vi "ValvulaUnitáriaV18.vi"() -> ()   [LabVIEW 2019]
uses:
  <vilib>/DAQmx/read.llb/DAQmx Read (Analog 1D DBL NChan 1Samp).vi
  <vilib>/DAQmx/read.llb/DAQmx Read (Analog 2D DBL NChan NSamp).vi
  <vilib>/DAQmx/create/channels.llb/DAQmx Create Channel (CO-Pulse Generation-Frequency).vi
  <vilib>/DAQmx/configure/timing.llb/DAQmx Timing (Implicit).vi
  <vilib>/DAQmx/configure/timing.llb/DAQmx Timing (Sample Clock).vi
  <vilib>/DAQmx/miscellaneous.llb/DAQmx Fill In Error Info.vi
  <vilib>/Analysis/NI_AALBase.lvlib
  <vilib>/Analysis/baseanly.llb/Mean (DBL).vi
  <resource>/objmgr/daqmx.rc
panel:
  out "Return from 0":bool
  out "Permanent regime":bool
  out "Samples saved":i32
  in  "Automático":bool
  in  "Duty Cycle %":dbl=50.0 min=5.0 max=50.0 step=1.0
  in  "Valvula 2":bool=TRUE
  in  "resetDaq":bool
  out "DAQ Rate":i32=100 min=1 max=10000 step=1
  in  "Samples per Cycle":i32=200 min=1 max=100000 step=1
  out "Motor stopping":bool
  out "Motor working":bool
  in  "Frequency":dbl=1.0 min=0.8 max=8.0 step=0.1
  out "CAME Frequency":dbl
  in  "Start Motor":bool
  out "StepMotorValueChanged":bool
  out "Cycles":i32
  in  "File Name":string="test"
  in  "?":enum32{"Page 1", "Page 2"}(tab)
  out "Torque":dbl(graph)
  out "Valve state signal":dbl[][](graph)
  out "Flowrate":dbl(graph)
  out "Pressures":dbl[][](graph)
  out "Displacements":dbl[][](graph)
  out "Indutive Sensor":dbl(graph)
  in  "Save aquisition":bool
  in  "File Path":path=path "G:/My Drive/MagChill/Sistema Hidráulico/6.Dados_Testes/2.Etapa_ii"
  in  "Stop":bool
  out "Stop operations":bool
  # "File Path"
  # "File name:"
  # "Eletrovalve/CAME\n       Frequency"
  # "Samples per Cycles"
  # "DAQ Rate"
  # "Cycles"
  # "Samples Saved"
  # "Write to File"
  # "Stop Program"
  # "CAME Operation"
  # "Start/Stop Motor\n(operation cycle)"
  # "CAME Frequency"
  # "Eletrovalve Operation"
  # "Start/Stop Eletrovalve\n     (operation cycle)"
  # "% Duty Cycle"
  # "On/Off Manual"
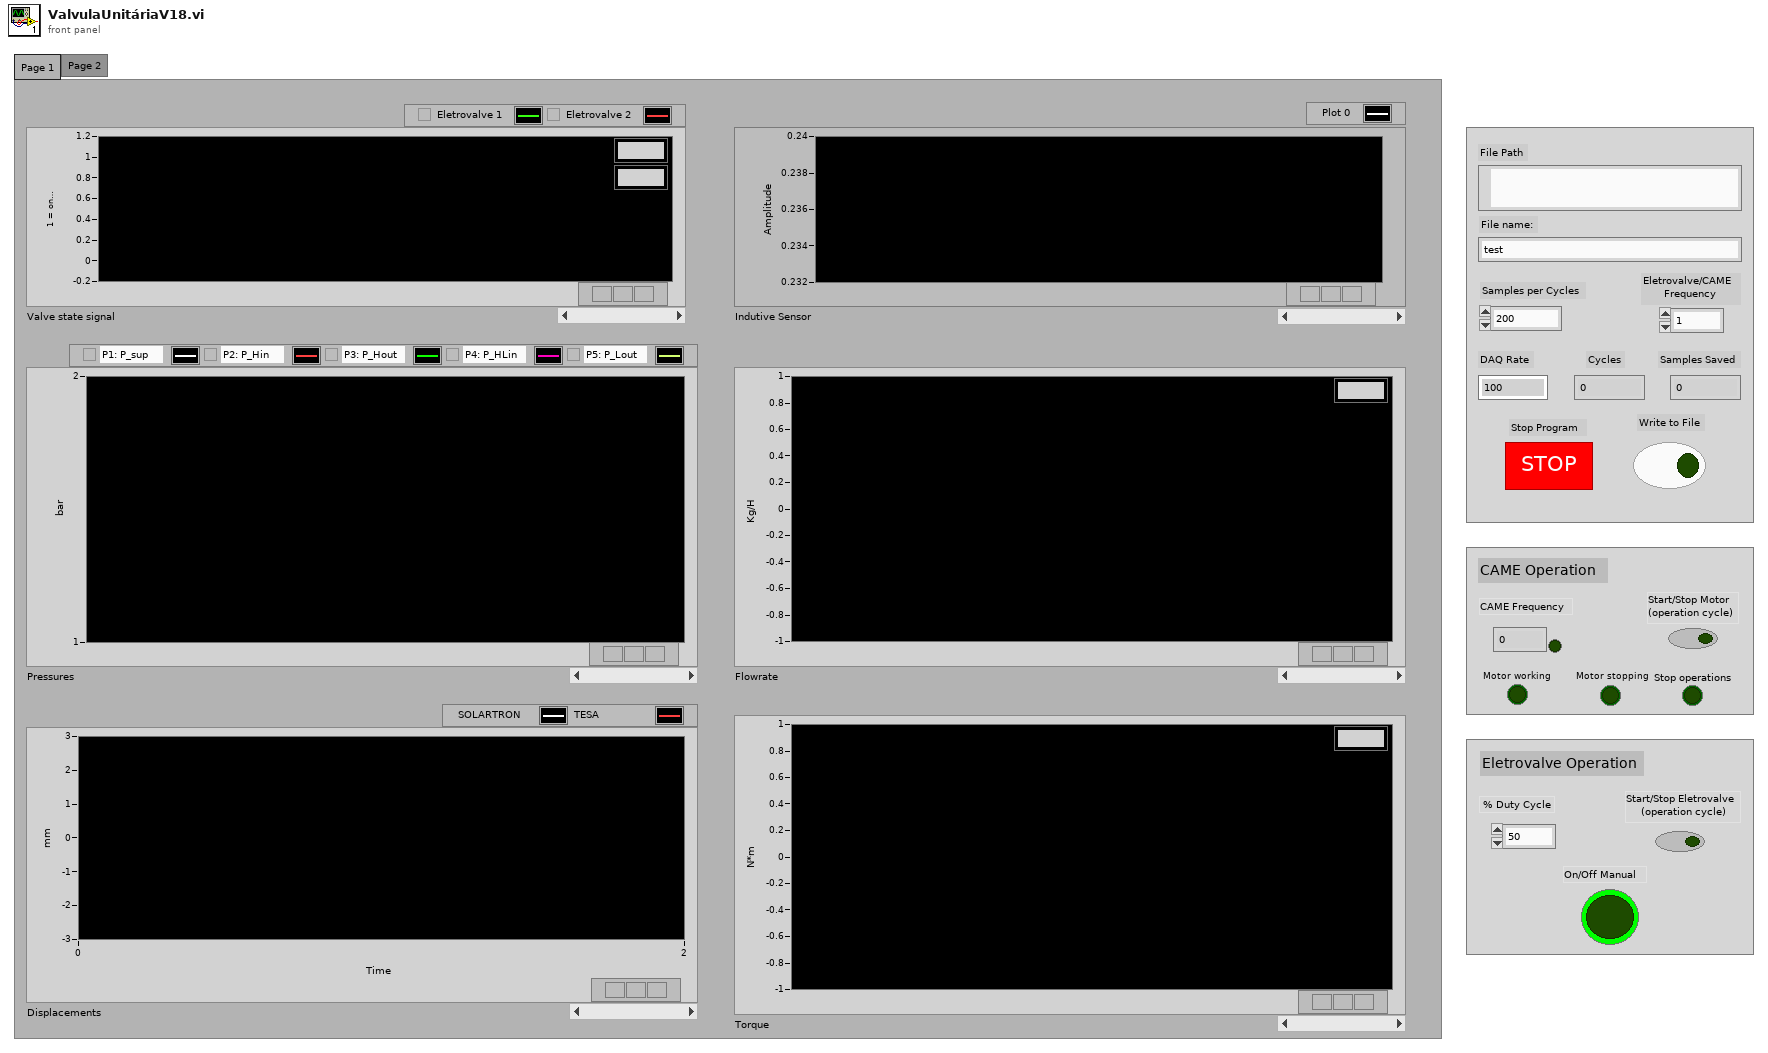
[diagram p1: front panel]
types:
  T1 = enum8{"Enabled", "Disabled", "Disabled and Grayed Out"}
  T2 = enum16{"open", "open or create", "create or replace", "create", "open (read only)"}
  T3 = cluster{"Automatico":bool, "Valvula":bool, "Duty cycle":dbl, "Stop":bool, "Frequencia":dbl}
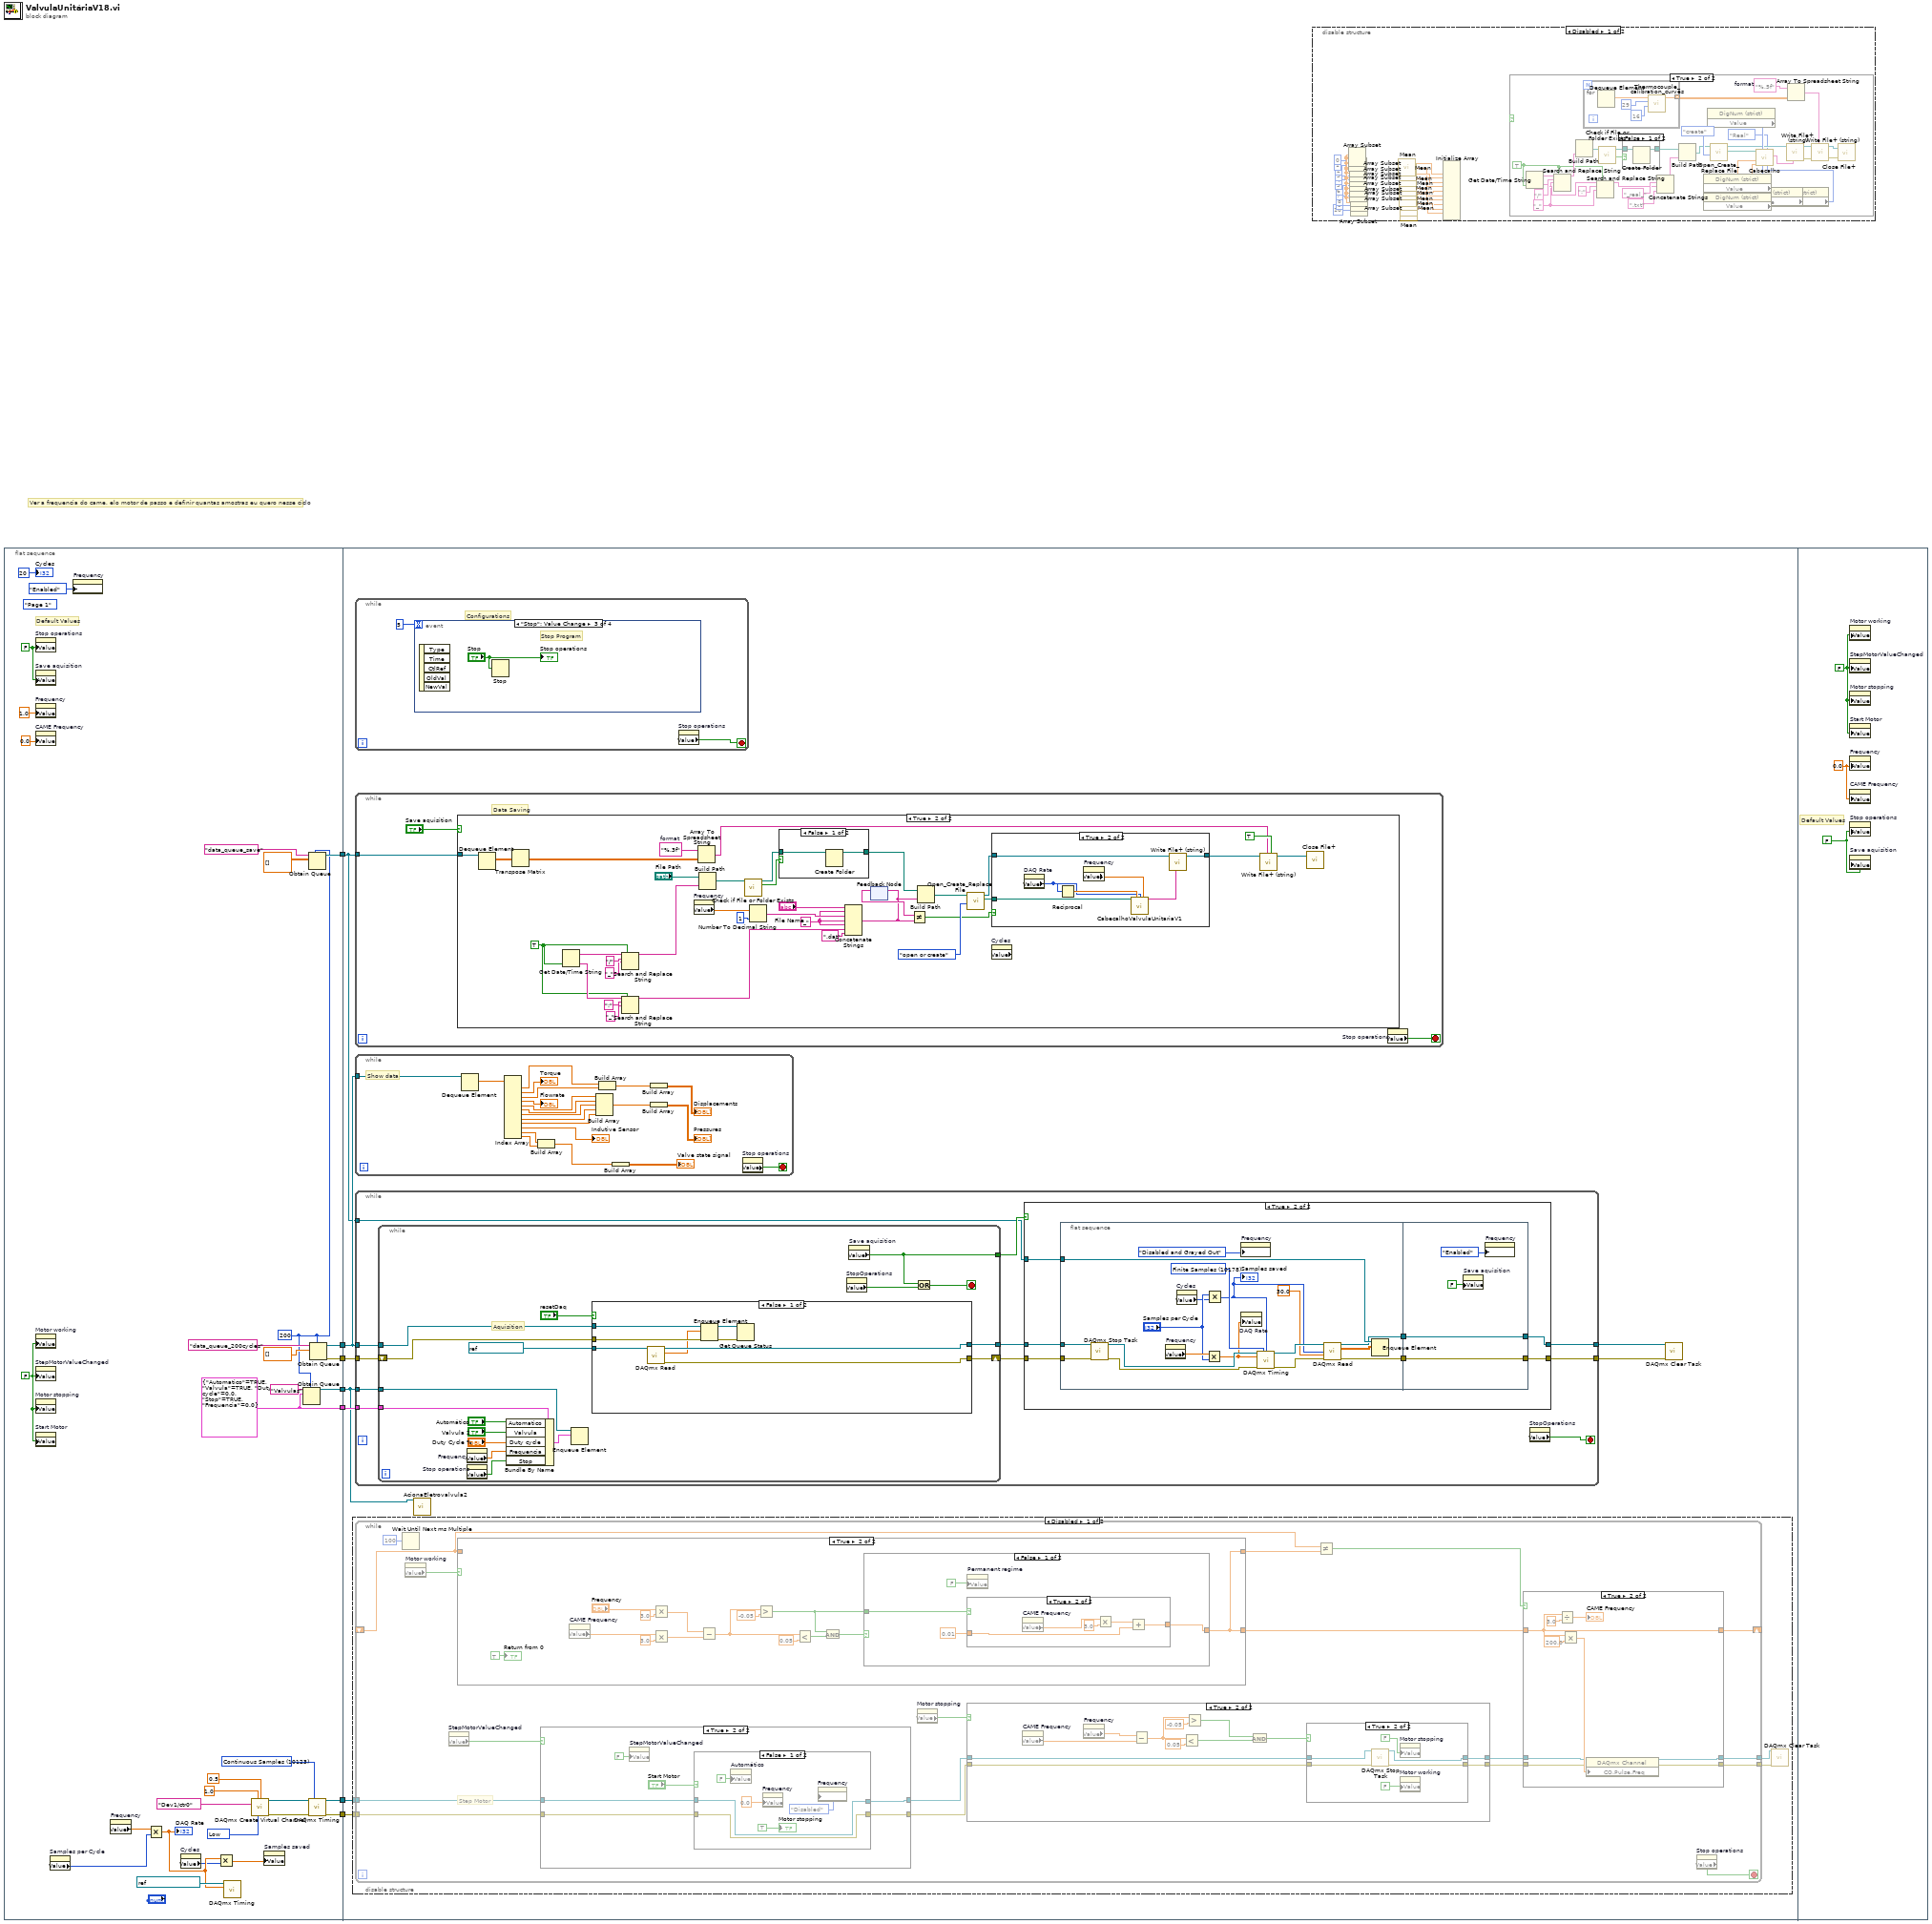
[diagram p0: block diagram]
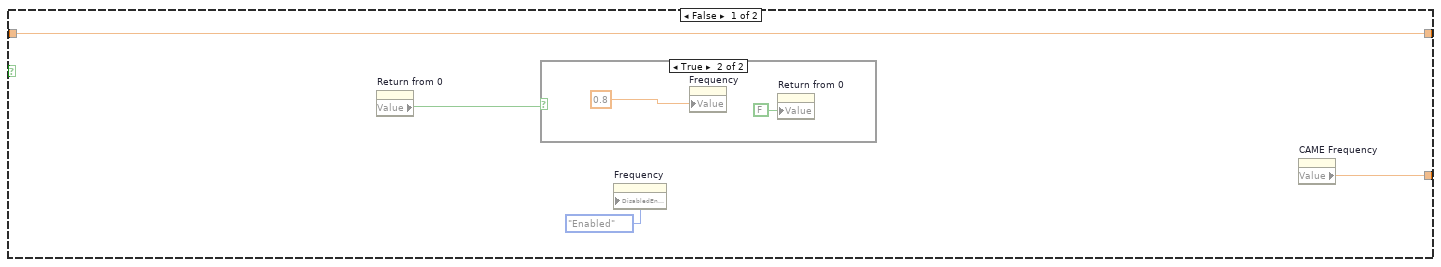
[diagram p4: hidden frame]
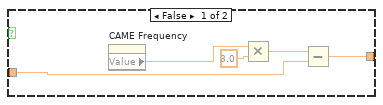
[diagram p6: hidden frame]
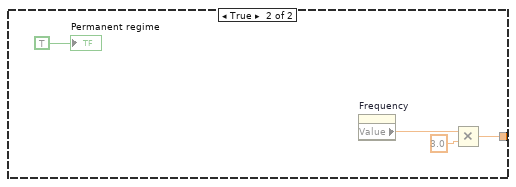
[diagram p7: hidden frame]
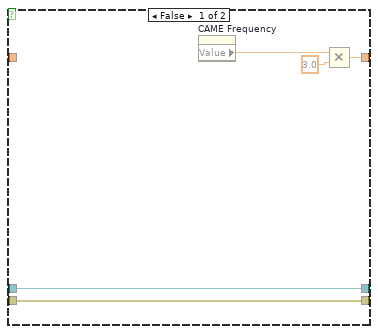
[diagram p8: hidden frame]
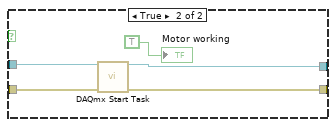
[diagram p10: hidden frame]
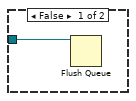
[diagram p12: hidden frame]
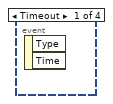
[diagram p15: hidden frame]
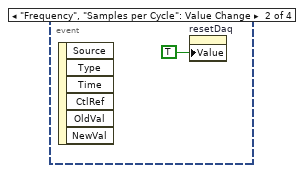
[diagram p16: hidden frame]
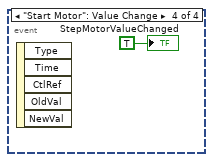
[diagram p17: hidden frame]
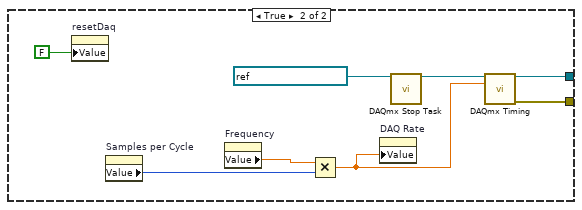
[diagram p19: hidden frame]
diagram:
  # "Ver a frequencia do came, elo motor de passo e definir quantas amostras eu quero nesse ciclo"
  n1 = flat-sequence {
    tunnel: [w39] -> w7
    tunnel: [w37] -> w6
    tunnel: [w28] -> w5
    tunnel: [w29] -> w4
    tunnel: [w24] -> w3
    tunnel: [w11] -> w2
    tunnel: [w10] -> w1
    tunnel: w7 -> [w43]
    tunnel: w6 -> [w48]
    tunnel: w5 -> [w46]
    tunnel: w4 -> [w47]
    tunnel: w3 -> [w42]
    tunnel: w2 -> [w40]
    tunnel: w1 -> [w41]
    frame #0 {
      w10 = T3 {"Automatico"=TRUE, "Valvula"=TRUE, "Duty cycle"=0.0, "Stop"=TRUE, "Frequencia"=0.0}
      w9 = 200 ("max queue size (-1, unlimited)")
      w26 = FALSE ("RestartOperations")
      w27 = FALSE
      w34 = 10123 items=["Finite Samples"=10178, "Continuous Samples"=10123, "Hardware Timed Single Point"=12522] ("sample mode")
      w30 = 10214 items=["High"=10192, "Low"=10214] ("idle state")
      (unwired) enum32{"Page 1", "Page 2"}."Page 1" ("Tab Control")
      # "Default Values"
      n2 = property on="Stop operations" class="Bool (strict)"("Value"=w26) -> ()  [unwired: 2 in, 2 out]
      n3 = property on="Save aquisition" class="Bool (strict)"("Value"=w26) -> ()  [unwired: 2 in, 2 out]
      n4 = property on="Frequency" class="DigNum (strict)"("Value"=1.0 ("SP CAME Frequency")) -> ()  [unwired: 2 in, 2 out]
      n5 = property on="CAME Frequency" class="DigNum (strict)"("Value"=0.0 ("CAME Frequency")) -> ()  [unwired: 2 in, 2 out]
      n6 = property on="Motor working" class="Bool (strict)"("Value"=w27) -> ()  [unwired: 2 in, 2 out]
      n7 = property on="StepMotorValueChanged" class="Bool (strict)"("Value"=w27) -> ()  [unwired: 2 in, 2 out]
      n8 = property on="Motor stopping" class="Bool (strict)"("Value"=w27) -> ()  [unwired: 2 in, 2 out]
      n9 = property on="Start Motor" class="Bool (strict)"("Value"=w27) -> ()  [unwired: 2 in, 2 out]
      n10 = property on="Samples per Cycle" class="DigNum (strict)"() -> ("Value"=w17:i32)  [unwired: 2 in, 2 out]
      n11 = property on="Frequency" class="DigNum (strict)"("DisabledEnum"=T1."Enabled" ("Disabled")) -> ()  [unwired: 2 in, 2 out]
      n12 = property on="Frequency" class="DigNum (strict)"() -> ("Value"=w21:dbl)  [unwired: 2 in, 2 out]
      n13 = Multiply(x=w21, y=w17) -> (x*y=w15:dbl)
      "DAQ Rate" <- w15
      n14 = property on="Cycles" class="DigNum (strict)"() -> ("Value"=w14:i32)  [unwired: 2 in, 2 out]
      n15 = Multiply(x=w15, y=w14) -> (x*y=w13:dbl)
      n16 = call-poly <vilib>:"DAQmx Timing.vi"("task/channels in"=refnum<k21> "AnalogInputs", "rate"=w15) -> ()  [unwired: 12 in, 2 out]
      n17 = call-poly <vilib>:"DAQmx Create Virtual Channel.vi"("frequency"=1.0, "duty cycle"=0.5, "counter"=tag "Dev1/ctr0", "idle state"=w30) -> ("task out"=w36:refnum<k21>, "error out"=w35:errorcluster)  [unwired: 10 in]
      n18 = property on="Samples saved" class="DigNum (strict)"("Value"=w13) -> ()  [unwired: 2 in, 2 out]
      n19 = Obtain Queue(max queue size (-1, unlimited)=w9, name (unnamed)="Valvulas", element data type=w10) -> (queue out=w11:refnum<queue>)  [unwired: 2 in, 2 out]
      n20 = Obtain Queue(max queue size (-1, unlimited)=w9, name (unnamed)="data_queue_save", element data type=dbl[][] [] ("data")) -> (queue out=w24:refnum<queue>)  [unwired: 2 in, 2 out]
      n21 = call-poly <vilib>:"DAQmx Timing.vi"("task/channels in"=w36, "sample mode"=w34, "error in"=w35) -> ("task out"=w29:refnum<k21>, "error out"=w28:errorcluster)  [unwired: 11 in]
      n22 = Obtain Queue(max queue size (-1, unlimited)=w9, name (unnamed)="data_queue_200cycles", element data type=dbl[] [] ("data")) -> (queue out=w39:refnum<queue>, error out=w37:errorcluster)  [unwired: 2 in, 1 out]
      "Cycles" <- 20 ("Cycles")
    }
    frame #1 {
      n23 = disable-structure shown="Disabled" {
        disable-tunnel: w47 -> [w52 _]
        disable-tunnel: w46 -> [w51 _]
        frame Disabled {
          n24 = while {
            tunnel: w52 -> [w70]
            tunnel: w51 -> [w69]
            shift-right: [w67] -> _
            shift-left: _ -> [w63]
            tunnel: [w55] -> w50
            tunnel: [w54] -> w49
            stop <- w53 stop-if-true
            # "Step Motor"
            n25 = Wait Until Next ms Multiple(millisecond multiple=u32 100) -> ()  [unwired: 1 out]
            n26 = property on="Motor working" class="Bool (strict)"() -> ("Value"=w66:bool)  [unwired: 2 in, 2 out]
            n27 = property on="StepMotorValueChanged" class="Bool (strict)"() -> ("Value"=w68:bool)  [unwired: 2 in, 2 out]
            n28 = case shown="True" w66 {
              tunnel: w63 -> [w96 _]
              tunnel: [w95 w108] -> w57
              tunnel: [w96 w108] -> w65
              frame False {
                n29 = property on="Return from 0" class="Bool (strict)"() -> ("Value"=w93:bool)  [unwired: 2 in, 2 out]
                n30 = case shown="True" w93 {
                  frame False {
                  }
                  frame True {
                    n31 = property on="Frequency" class="DigNum (strict)"("Value"=0.8 ("SP Frequency")) -> ()  [unwired: 2 in, 2 out]
                    n32 = property on="Return from 0" class="Bool (strict)"("Value"=FALSE ("Return from 0")) -> ()  [unwired: 2 in, 2 out]
                  }
                }
                n33 = property on="Frequency" class="DigNum (strict)"("DisabledEnum"=T1."Enabled" ("Disabled")) -> ()  [unwired: 2 in, 2 out]
                n34 = property on="CAME Frequency" class="DigNum (strict)"() -> ("Value"=w95:dbl)  [unwired: 2 in, 2 out]
              }
              frame True {
                n35 = property on="CAME Frequency" class="DigNum (strict)"() -> ("Value"=w103:dbl)  [unwired: 2 in, 2 out]
                n36 = Multiply(x="Frequency", y=3.0) -> (x*y=w104:dbl)
                n37 = Multiply(x=w103, y=3.0) -> (x*y=w101:dbl)
                n38 = Subtract(x=w104, y=w101) -> (x-y=w106:dbl)
                n39 = Greater?(x=w106, y=-0.05) -> (0:w107:bool)
                n40 = Less?(x=w106, y=0.05) -> (x < y?=w110:bool)
                n41 = And(x=w107, y=w110) -> (x .and. y?=w109:bool)
                n42 = case shown="False" w109 {
                  tunnel: [w115 w130] -> w108
                  tunnel: w107 -> [w116 _]
                  frame False {
                    n43 = property on="Permanent regime" class="Bool (strict)"("Value"=FALSE ("Permanent regime")) -> ()  [unwired: 2 in, 2 out]
                    n44 = case shown="True" w116 {
                      tunnel: [w121 w126] -> w115
                      tunnel: 0.01 ("y") -> [w120 w125]
                      frame False {
                        n45 = property on="CAME Frequency" class="DigNum (strict)"() -> ("Value"=w119:dbl)  [unwired: 2 in, 2 out]
                        n46 = Multiply(x=w119, y=3.0) -> (x*y=w117:dbl)
                        n47 = Subtract(x=w117, y=w120) -> (x-y=w121:dbl)
                      }
                      frame True {
                        n48 = property on="CAME Frequency" class="DigNum (strict)"() -> ("Value"=w124:dbl)  [unwired: 2 in, 2 out]
                        n49 = Multiply(x=w124, y=3.0) -> (x*y=w122:dbl)
                        n50 = Add(x=w122, y=w125) -> (x+y=w126:dbl)
                      }
                    }
                  }
                  frame True {
                    n51 = property on="Frequency" class="DigNum (strict)"() -> ("Value"=w129:dbl)  [unwired: 2 in, 2 out]
                    n52 = Multiply(x=w129, y=3.0) -> (x*y=w130:dbl)
                    "Permanent regime" <- TRUE ("Permanent regime")
                  }
                }
                "Return from 0" <- TRUE ("Return from 0")
              }
            }
            n53 = case shown="True" w68 {
              tunnel: w70 -> [w146 w151]
              tunnel: w69 -> [w145 w150]
              tunnel: [w146 w147] -> w61
              tunnel: [w145 w152] -> w60
              frame False {
              }
              frame True {
                n54 = property on="StepMotorValueChanged" class="Bool (strict)"("Value"=FALSE) -> ()  [unwired: 2 in, 2 out]
                n55 = case shown="False" "Start Motor" {
                  tunnel: [w157 w163] -> w147
                  tunnel: [w156 w162] -> w152
                  tunnel: w151 -> [w157 w161]
                  tunnel: w150 -> [w156 w160]
                  frame False {
                    n56 = property on="Automático" class="Bool (strict)"("Value"=FALSE ("Automático")) -> ()  [unwired: 2 in, 2 out]
                    n57 = property on="Frequency" class="DigNum (strict)"("Value"=0.0 ("SP Frequency")) -> ()  [unwired: 2 in, 2 out]
                    n58 = property on="Frequency" class="DigNum (strict)"("DisabledEnum"=T1."Disabled" ("Disabled")) -> ()  [unwired: 2 in, 2 out]
                    "Motor stopping" <- TRUE ("Motor stopping")
                  }
                  frame True {
                    n59 = call <vilib>:"DAQmx Start Task.vi"("task/channels in"=w161, "error in"=w160) -> ("task out"=w163:refnum<k21>, "error out"=w162:errorcluster)  [unwired: 12 in]
                    "Motor working" <- TRUE ("Motor working")
                  }
                }
              }
            }
            n60 = property on="Motor stopping" class="Bool (strict)"() -> ("Value"=w62:bool)  [unwired: 2 in, 2 out]
            n61 = case shown="True" w62 {
              tunnel: w61 -> [w72 w78]
              tunnel: w60 -> [w71 w77]
              tunnel: [w72 w76] -> w59
              tunnel: [w71 w75] -> w58
              frame False {
              }
              frame True {
                n62 = property on="CAME Frequency" class="DigNum (strict)"() -> ("Value"=w73:dbl)  [unwired: 2 in, 2 out]
                n63 = property on="Frequency" class="DigNum (strict)"() -> ("Value"=w80:dbl)  [unwired: 2 in, 2 out]
                n64 = Subtract(x=w80, y=w73) -> (x-y=w83:dbl)
                n65 = Less?(x=w83, y=0.05) -> (x < y?=w82:bool)
                n66 = Greater?(x=w83, y=-0.05) -> (0:w81:bool)
                n67 = And(x=w81, y=w82) -> (x .and. y?=w79:bool)
                n68 = case shown="True" w79 {
                  tunnel: w78 -> [w86 w92]
                  tunnel: w77 -> [w85 w91]
                  tunnel: [w86 w90] -> w76
                  tunnel: [w85 w89] -> w75
                  frame False {
                  }
                  frame True {
                    n69 = call <vilib>:"DAQmx Stop Task.vi"("task/channels in"=w92, "error in"=w91) -> ("task out"=w90:refnum<k21>, "error out"=w89:errorcluster)  [unwired: 12 in]
                    n70 = property on="Motor stopping" class="Bool (strict)"("Value"=FALSE ("Motor stopping")) -> ()  [unwired: 2 in, 2 out]
                    n71 = property on="Motor working" class="Bool (strict)"("Value"=FALSE ("Motor working")) -> ()  [unwired: 2 in, 2 out]
                  }
                }
              }
            }
            n72 = Not Equal?(x=w63, y=w65) -> (x != y?=w64:bool)
            n73 = case shown="True" w64 {
              tunnel: [w135 w144] -> w55
              tunnel: [w134 w143] -> w54
              tunnel: w57 -> [_ w137]
              tunnel: [w131 w137] -> w67
              tunnel: w59 -> [w135 w140]
              tunnel: w58 -> [w134 w139]
              frame False {
                n74 = property on="CAME Frequency" class="DigNum (strict)"() -> ("Value"=w133:dbl)  [unwired: 2 in, 2 out]
                n75 = Multiply(x=w133, y=3.0) -> (x*y=w131:dbl)
              }
              frame True {
                n76 = Divide(x=w137, y=3.0) -> (x/y=→"CAME Frequency":dbl)
                n77 = Multiply(x=w137, y=200.0) -> (x*y=w141:dbl)
                n78 = property class="DAQmx Channel"(reference=w140, error in=w139, "CO.Pulse.Freq"=w141) -> (reference out=w144:refnum<k21>, error out=w143:errorcluster)
              }
            }
            n79 = property on="Stop operations" class="Bool (strict)"() -> ("Value"=w53:bool)  [unwired: 2 in, 2 out]
          }
          n80 = call <vilib>:"DAQmx Clear Task.vi"("task in"=w50, "error in"=w49) -> ()  [unwired: 13 in, 1 out]
        }
        frame Enabled {
        }
      }
      n81 = while {
        stop <- w235 stop-if-true
        # "Configurations"
        n82 = event shown="[2] \"Stop\": Value Change" {
          selector: _ -> [_ _ _ _]
          dyn-events: _ -> [_ _ _ _]
          timeout: 5 -> [_ _ _ _]
          event Timeout {
            n83 = event-data() -> ()  [unwired: 1 in, 2 out]
          }
          event "Frequency", "Samples per Cycle": Value Change {
            n84 = event-data() -> ()  [unwired: 1 in, 6 out]
            n85 = property on="resetDaq" class="Bool (strict)"("Value"=TRUE ("resetDaq")) -> ()  [unwired: 2 in, 2 out]
          }
          event "Stop": Value Change {
            # "Stop Program"
            n86 = event-data() -> ()  [unwired: 1 in, 5 out]
            n87 = Stop(stop? (T)="Stop") -> ()
            "Stop operations" <- "Stop"
          }
          event "Start Motor": Value Change {
            n88 = event-data() -> ()  [unwired: 1 in, 5 out]
            "StepMotorValueChanged" <- TRUE
          }
        }
        n89 = property on="Stop operations" class="Bool (strict)"() -> ("Value"=w235:bool)  [unwired: 2 in, 2 out]
      }
      n90 = while {
        tunnel: w42 -> [w165]
        stop <- w166 stop-if-true
        # "Data Saving"
        n91 = case shown="True" "Save aquisition" {
          tunnel: w165 -> [w167 w202]
          frame False {
            n92 = Flush Queue(queue=w167) -> ()  [unwired: 1 in, 3 out]
          }
          frame True {
            w171 = "_" ("replace string (\"\")")
            w172 = TRUE ("want seconds? (F)")
            w201 = "%.3f"  # format
            n93 = Dequeue Element(queue=w202) -> (element=w170:dbl[][])  [unwired: 2 in, 3 out]
            n94 = Transpose Matrix(1:w170) -> (0:w168:dbl[][])
            n95 = Get Date/Time String(want seconds? (F)=w172) -> (date string=w195:string, time string=w176:string)  [unwired: 2 out]
            n96 = Search and Replace String(replace all?=w172, input string=w195, search string="/" ("string"), replace string="_" ("replace string (\"\")")) -> (result string=w194:string)  [unwired: 4 in, 3 out]
            n97 = Search and Replace String(replace all?=w172, input string=w176, search string=":" ("string"), replace string="_" ("replace string (\"\")")) -> (result string=w173:string)  [unwired: 4 in, 3 out]
            n98 = property on="Frequency" class="DigNum (strict)"() -> ("Value"=w182:dbl)  [unwired: 2 in, 2 out]
            n99 = Array To Spreadsheet String(array=w168, 3:w201) -> (spreadsheet string=w169:string)  [unwired: 1 out]
            n100 = Build Path(base path="File Path", name or relative path=w194) -> (appended path=w199:path)
            n101 = call <vilib>:"Check if File or Folder Exists.vi"("path"=w199) -> ("file or folder exists?"=w198:bool, "dup path"=w197:path)  [unwired: 8 in, 1 out]
            n102 = Number To Decimal String(number=w182, width (-)=i16 1) -> (decimal integer string=w184:string)
            n103 = case shown="False" w198 {
              tunnel: w197 -> [w212 w213]
              tunnel: [w211 w213] -> w190
              frame False {
                n104 = Create Folder(path (use dialog)=w212) -> (created path=w211:path)  [unwired: 2 in, 2 out]
              }
              frame True {
              }
            }
            n105 = Concatenate Strings("File Name", w171, w184, w171, w171, w173, ".dat" ("string")) -> (w179:string)
            n106 = feedback #1() -> (w180:string)  [unwired: 1 in]
            n107 = feedback-in #1(w179) -> ()
            n108 = Not Equal?(x=w180, y=w179) -> (x != y?=w181:bool)
            n109 = Build Path(base path=w190, name or relative path=w179) -> (appended path=w191:path)
            n110 = call <vilib>:"Open_Create_Replace File.vi"("function (open:0)"=T2."open or create", "file path"=w191) -> ("new file path"=w187:path, "refnum"=w188:refnum<file>)  [unwired: 4 in, 4 out]
            n111 = case shown="True" w181 {
              tunnel: w187 -> [_ w205]
              tunnel: w188 -> [w203 w210]
              tunnel: [w203 w209] -> w189
              frame False {
              }
              frame True {
                n112 = property on="DAQ Rate" class="DigNum (strict)"() -> ("Value"=w207:i32)  [unwired: 2 in, 2 out]
                n113 = Reciprocal(x=w207) -> (1/x=w208:dbl)
                n114 = property on="Frequency" class="DigNum (strict)"() -> ("Value"=w206:dbl)  [unwired: 2 in, 2 out]
                n115 = call "CabecalhoValvulaUnitariaV1.vi"("Output File"=w205, "Delta t"=w208, "DAQ Rate"=w207, "SP CAME Frequency"=w206) -> ("data file"=w204:string)  [unwired: 11 in]
                n116 = call <vilib>:"Write File+ (string).vi"("string"=w204, "refnum"=w210) -> ("dup refnum"=w209:refnum<file>)  [unwired: 4 in, 3 out]
              }
            }
            n117 = property on="Cycles" class="DigNum (strict)" props=["Value"]() -> ()  [unwired: 2 in, 3 out]
            n118 = call <vilib>:"Write File+ (string).vi"("convert eol? (no:F)"=TRUE, "string"=w169, "refnum"=w189) -> ("dup refnum"=w196:refnum<file>)  [unwired: 3 in, 3 out]
            n119 = call <vilib>:"Close File+.vi"("refnum"=w196) -> ()  [unwired: 2 in, 5 out]
          }
        }
        n120 = property on="Stop operations" class="Bool (strict)"() -> ("Value"=w166:bool)  [unwired: 2 in, 2 out]
      }
      n121 = while {
        tunnel: w43 -> [w222]
        stop <- w220 stop-if-true
        # "Show data"
        n122 = Dequeue Element(queue=w222) -> (element=w221:dbl[])  [unwired: 1 in, 4 out]
        n123 = Index Array(array=w221) -> (element #1=w233:dbl, element #2=→"Torque":dbl, element #3=w234:dbl, element #4=→"Flowrate":dbl, element #5=w232:dbl, element #6=w226:dbl, element #7=w225:dbl, element #8=w224:dbl, element #9=w223:dbl, element #10=→"Indutive Sensor":dbl, element #11=w217:dbl, element #12=w216:dbl)  [unwired: 12 in]
        n124 = Build Array(w217, w216) -> (w215:dbl[])
        n125 = Build Array(w232, w226, w225, w224, w223) -> (w230:dbl[])
        n126 = Build Array(w233, w234) -> (w228:dbl[])
        n127 = Build Array(w215) -> (→"Valve state signal":dbl[][])
        n128 = Build Array(w228) -> (→"Displacements":dbl[][])
        n129 = Build Array(w230) -> (→"Pressures":dbl[][])
        n130 = property on="Stop operations" class="Bool (strict)"() -> ("Value"=w220:bool)  [unwired: 2 in, 2 out]
      }
      n131 = while {
        tunnel: [w243] -> w45
        tunnel: [w242] -> w44
        tunnel: w43 -> [w250]
        tunnel: w48 -> [w249]
        tunnel: w42 -> [w244]
        tunnel: w40 -> [w241]
        tunnel: w41 -> [w240]
        stop <- w248 stop-if-true
        n132 = while {
          tunnel: [w298] -> w246
          tunnel: w250 -> [w295]
          shift-right: [w297] -> w245
          shift-left: w249 -> [w294]
          tunnel: [w290] -> w247
          tunnel: w241 -> [w283]
          tunnel: w240 -> [w289]
          stop <- w291 stop-if-true
          # "Aquisition"
          n133 = property on="Frequency" class="DigNum (strict)"() -> ("Value"=w285:dbl)  [unwired: 2 in, 2 out]
          n134 = property on="Stop operations" class="Bool (strict)"() -> ("Value"=w284:bool)  [unwired: 2 in, 2 out]
          n135 = Bundle By Name(cluster=w289, "Automatico"="Automático", "Valvula"="Valvula 2", "Duty cycle"="Duty Cycle %", "Frequencia"=w285, "Stop"=w284) -> (w282:T3)
          n136 = Enqueue Element(queue=w283, element=w282) -> ()  [unwired: 2 in, 3 out]
          n137 = case shown="False" "resetDaq" {
            tunnel: [w306 w311] -> w298
            tunnel: [w305 w310] -> w297
            tunnel: refnum<k21> "AnalogInputs" ("DAQmx Task Name") -> [w304 _]
            tunnel: w295 -> [w303 _]
            tunnel: w294 -> [w301 _]
            frame False {
              n138 = call-poly <vilib>:"DAQmx Read.vi"("task/channels in"=w304) -> ("task out"=w306:refnum<k21>, "data"=w299:dbl[], "error out"=w305:errorcluster)  [unwired: 12 in]
              n139 = Enqueue Element(queue=w303, element=w299, error in (no error)=w301) -> (queue out=w302:refnum<queue>, error out=w300:errorcluster)  [unwired: 1 in, 1 out]
              n140 = Get Queue Status(queue=w302, error in (no error)=w300) -> ()  [unwired: 1 in, 8 out]
            }
            frame True {
              n141 = property on="resetDaq" class="Bool (strict)"("Value"=FALSE ("resetDaq")) -> ()  [unwired: 2 in, 2 out]
              n142 = property on="Samples per Cycle" class="DigNum (strict)"() -> ("Value"=w307:i32)  [unwired: 2 in, 2 out]
              n143 = property on="Frequency" class="DigNum (strict)"() -> ("Value"=w313:dbl)  [unwired: 2 in, 2 out]
              n144 = Multiply(x=w313, y=w307) -> (x*y=w308:dbl)
              n145 = property on="DAQ Rate" class="DigNum (strict)"("Value"=w308) -> ()  [unwired: 2 in, 2 out]
              n146 = call <vilib>:"DAQmx Stop Task.vi"("task/channels in"=refnum<k21> "AnalogInputs") -> ("task out"=w314:refnum<k21>)  [unwired: 13 in, 1 out]
              n147 = call-poly <vilib>:"DAQmx Timing.vi"("task/channels in"=w314, "rate"=w308) -> ("task out"=w311:refnum<k21>, "error out"=w310:errorcluster)  [unwired: 12 in]
            }
          }
          n148 = property on="StopOperations" class="Bool (strict)"() -> ("Value"=w292:bool)  [unwired: 2 in, 2 out]
          n149 = property on="Save aquisition" class="Bool (strict)"() -> ("Value"=w290:bool)  [unwired: 2 in, 2 out]
          n150 = Or(x=w290, y=w292) -> (x .or. y?=w291:bool)
        }
        n151 = case shown="True" w247 {
          tunnel: w246 -> [w252 w259]
          tunnel: w245 -> [w251 w258]
          tunnel: w244 -> [_ w257]
          tunnel: [w252 w255] -> w243
          tunnel: [w251 w253] -> w242
          frame False {
          }
          frame True {
            n152 = flat-sequence {
              tunnel: w259 -> [w277]
              tunnel: w258 -> [w276]
              tunnel: w257 -> [w270]
              tunnel: [w268] -> w256
              tunnel: [w267] -> w254
              tunnel: w256 -> [w279]
              tunnel: [w279] -> w255
              tunnel: w254 -> [w278]
              tunnel: [w278] -> w253
              frame #0 {
                w274 = 10178 items=["Finite Samples"=10178, "Continuous Samples"=10123, "Hardware Timed Single Point"=12522] ("sample mode")
                n153 = call <vilib>:"DAQmx Stop Task.vi"("task/channels in"=w277, "error in"=w276) -> ("task out"=w275:refnum<k21>, "error out"=w271:errorcluster)  [unwired: 12 in]
                n154 = property on="Frequency" class="DigNum (strict)"() -> ("Value"=w266:dbl)  [unwired: 2 in, 2 out]
                n155 = property on="Cycles" class="DigNum (strict)"() -> ("Value"=w261:i32)  [unwired: 2 in, 2 out]
                n156 = Multiply(x=w266, y="Samples per Cycle") -> (x*y=w262:dbl)
                n157 = Multiply(x="Samples per Cycle", y=w261) -> (x*y=w260:i32)
                "Samples saved" <- w260
                n158 = property on="Frequency" class="DigNum (strict)"("DisabledEnum"=T1."Disabled and Grayed Out" ("Disabled")) -> ()  [unwired: 2 in, 2 out]
                n159 = property on="DAQ Rate" class="DigNum (strict)"("Value"=w262) -> ()  [unwired: 2 in, 2 out]
                n160 = call-poly <vilib>:"DAQmx Timing.vi"("task/channels in"=w275, "sample mode"=w274, "samples per channel"=w260, "rate"=w262, "error in"=w271) -> ("task out"=w273:refnum<k21>, "error out"=w272:errorcluster)  [unwired: 9 in]
                n161 = call-poly <vilib>:"DAQmx Read.vi"("task/channels in"=w273, "number of samples per channel"=w260, "timeout"=30.0, "error in"=w272) -> ("task out"=w268:refnum<k21>, "data"=w269:dbl[][], "error out"=w267:errorcluster)  [unwired: 9 in]
                n162 = Enqueue Element(queue=w270, element=w269) -> ()  [unwired: 2 in, 3 out]
              }
              frame #1 {
                n163 = property on="Save aquisition" class="Bool (strict)"("Value"=FALSE ("Save aquisition")) -> ()  [unwired: 2 in, 2 out]
                n164 = property on="Frequency" class="DigNum (strict)"("DisabledEnum"=T1."Enabled" ("Disabled")) -> ()  [unwired: 2 in, 2 out]
              }
            }
          }
        }
        n165 = property on="StopOperations" class="Bool (strict)"() -> ("Value"=w248:bool)  [unwired: 2 in, 2 out]
      }
      n166 = call "AcionaEletrovalvula2.vi"("queue Variaveis"=w40) -> ()  [unwired: 11 in]
      n167 = call <vilib>:"DAQmx Clear Task.vi"("task in"=w45, "error in"=w44) -> ()  [unwired: 13 in, 1 out]
    }
    frame #2 {
      w315 = FALSE ("RestartOperations")
      w316 = 0.0 ("Frequency SM")
      w317 = FALSE
      # "Default Values"
      n168 = property on="Motor working" class="Bool (strict)"("Value"=w317) -> ()  [unwired: 2 in, 2 out]
      n169 = property on="StepMotorValueChanged" class="Bool (strict)"("Value"=w317) -> ()  [unwired: 2 in, 2 out]
      n170 = property on="Motor stopping" class="Bool (strict)"("Value"=w317) -> ()  [unwired: 2 in, 2 out]
      n171 = property on="Start Motor" class="Bool (strict)"("Value"=w317) -> ()  [unwired: 2 in, 2 out]
      n172 = property on="Frequency" class="DigNum (strict)"("Value"=w316) -> ()  [unwired: 2 in, 2 out]
      n173 = property on="CAME Frequency" class="DigNum (strict)"("Value"=w316) -> ()  [unwired: 2 in, 2 out]
      n174 = property on="Stop operations" class="Bool (strict)"("Value"=w315) -> ()  [unwired: 2 in, 2 out]
      n175 = property on="Save aquisition" class="Bool (strict)"("Value"=w315) -> ()  [unwired: 2 in, 2 out]
    }
  }
  n176 = disable-structure shown="Disabled" {
    frame Disabled {
      (unwired) 8 ("index")
      (unwired) 6 ("index")
      (unwired) 2 ("index")
      n177 = Array Subset(index=0) -> (array=w327:dbl[])  [unwired: 1 in, 1 out]
      n178 = Array Subset(array=w327, index=1) -> ()  [unwired: 1 in, 1 out]
      n179 = Array Subset(array=w327) -> ()  [unwired: 2 in, 1 out]
      n180 = Array Subset(array=w327, index=3) -> ()  [unwired: 1 in, 1 out]
      n181 = Array Subset(array=w327, index=4) -> ()  [unwired: 1 in, 1 out]
      n182 = Array Subset(array=w327, index=5) -> ()  [unwired: 1 in, 1 out]
      n183 = Array Subset(array=w327) -> ()  [unwired: 2 in, 1 out]
      n184 = Array Subset(array=w327, index=7) -> ()  [unwired: 1 in, 1 out]
      n185 = Array Subset(array=w327) -> ()  [unwired: 2 in, 1 out]
      n186 = Array Subset(array=w327, index=9) -> ()  [unwired: 1 in, 1 out]
      n187 = Array Subset(array=w327, index=10) -> (w326:void[])  [unwired: 1 in]
      n188 = call-poly <vilib>:"Mean.vi"() -> ("mean"=w328:dbl)  [unwired: 1 in, 1 out]
      n189 = call-poly <vilib>:"Mean.vi"() -> ("mean"=w329:dbl)  [unwired: 1 in, 1 out]
      n190 = call-poly <vilib>:"Mean.vi"() -> ("mean"=w330:dbl)  [unwired: 1 in, 1 out]
      n191 = call-poly <vilib>:"Mean.vi"() -> ("mean"=w332:dbl)  [unwired: 1 in, 1 out]
      n192 = call-poly <vilib>:"Mean.vi"() -> ("mean"=w331:dbl)  [unwired: 1 in, 1 out]
      n193 = call-poly <vilib>:"Mean.vi"() -> ("mean"=w333:dbl)  [unwired: 1 in, 1 out]
      n194 = call-poly <vilib>:"Mean.vi"() -> ("mean"=w334:dbl)  [unwired: 1 in, 1 out]
      n195 = call-poly <vilib>:"Mean.vi"() -> ("mean"=w335:dbl)  [unwired: 1 in, 1 out]
      n196 = call-poly <vilib>:"Mean.vi"() -> ("mean"=w337:dbl)  [unwired: 1 in, 1 out]
      n197 = call-poly <vilib>:"Mean.vi"() -> ("mean"=w336:dbl)  [unwired: 1 in, 1 out]
      n198 = Initialize Array(w328, w329, w330, w331, w332, w333, w334, w335, w336, w337) -> ()  [unwired: 2 in, 1 out]
      n199 = case shown="True" {
        selector: _ -> [_ _]
        frame False {
        }
        frame True {
          w344 = "%.5f"  # format
          w338 = TRUE ("replace all? (F)")
          w352 = "_" ("replace string (\"\")")
          n200 = Get Date/Time String(want seconds? (F)=w338) -> (date string=w359:string, time string=w354:string)  [unwired: 2 out]
          n201 = Search and Replace String(replace all?=w338, input string=w359, search string="/", replace string=w352) -> (result string=w358:string)  [unwired: 4 in, 3 out]
          n202 = Build Path(name or relative path=w358) -> (base path=w361:path, appended path=w357:path)
          n203 = for {
            tunnel: [w376] -> w345 mode=indexing
            n204 = Dequeue Element() -> (element=w375:dbl[])  [unwired: 3 in, 3 out]
            n205 = call "Thermocouple_calibration_curves.vi"("split length 2"=16, "split length 1"=29, "Array in"=w375) -> ("Array out"=w376:dbl[])  [unwired: 8 in]
          }
          n206 = Search and Replace String(replace all?=w338, input string=w354, search string=":", replace string=w352) -> (result string=w350:string)  [unwired: 4 in, 3 out]
          n207 = call <vilib>:"Check if File or Folder Exists.vi"("path"=w357) -> ("file or folder exists?"=w356:bool, "dup path"=w355:path)  [unwired: 8 in, 1 out]
          n208 = case shown="False" w356 {
            tunnel: w355 -> [w373 w374]
            tunnel: [w372 w374] -> w348
            frame False {
              n209 = Create Folder(path (use dialog)=w373) -> (created path=w372:path)  [unwired: 2 in, 2 out]
            }
            frame True {
            }
          }
          n210 = Concatenate Strings("_real_" ("string"), w350, ".txt" ("string")) -> (w347:string)  [unwired: 1 in]
          n211 = Build Path(base path=w348, name or relative path=w347) -> (appended path=w346:path)
          n212 = property on="Property Node" class="DigNum (strict)"() -> ("Value"=w368:dbl)  [unwired: 2 in, 2 out]
          n213 = property on="Property Node" class="DigNum (strict)"() -> ("Value"=w369:dbl)  [unwired: 2 in, 2 out]
          n214 = property on="Property Node" class="DigNum (strict)"() -> ("Value"=w367:i32)  [unwired: 2 in, 2 out]
          n215 = call <vilib>:"Open_Create_Replace File.vi"("function (open:0)"=T2."create", "file path"=w346) -> ("new file path"=w365:path, "refnum"=w364:refnum<file>)  [unwired: 4 in, 4 out]
          n216 = property on="Property Node" class="DigNum (strict)"() -> ("Value"=w370:i32)  [unwired: 2 in, 2 out]
          n217 = property on="Property Node" class="DigNum (strict)"() -> ("Value"=w371:i32)  [unwired: 2 in, 2 out]
          n218 = call "Cabecalho.vi"("Hot Fan"=w371, "Type"=enum16{"Mean", "Real"}."Real", "Cold Fan"=w370, "Rot Pump"=w367, "FB"=w369, "f AMR"=w368, "Output File"=w365) -> ("data file"=w366:string)  [unwired: 4 in]
          n219 = call <vilib>:"Write File+ (string).vi"("string"=w366, "refnum"=w364) -> ("error out"=w343:errorcluster, "dup refnum"=w342:refnum<file>)  [unwired: 4 in, 2 out]
          n220 = Array To Spreadsheet String(array=w345, 3:w344) -> (spreadsheet string=w341:string)  [unwired: 1 out]
          n221 = call <vilib>:"Write File+ (string).vi"("string"=w341, "error in (no error)"=w343, "refnum"=w342) -> ("error out"=w339:errorcluster, "dup refnum"=w340:refnum<file>)  [unwired: 3 in, 2 out]
          n222 = call <vilib>:"Close File+.vi"("error in (no error)"=w339, "refnum"=w340) -> ()  [unwired: 1 in, 5 out]
        }
      }
    }
    frame Enabled {
    }
  }
